vi "HandleScore.vi"(8 "error in (no error)":errorcluster, 11 "Pong in":refnum<class "Pong.lvclass">) -> (0 "error out":errorcluster, 3 "Pong out":refnum<class "Pong.lvclass">)   [LabVIEW 2019, in "RT_Game.lvlib" / "Pong.lvclass"]
uses:
  Pong.lvclass
  C:/Users/FreshBob/Dropbox/VIs/myRIO_GameConsole/RT/RT_Game/Game/Game.lvclass
  Game/Coordinate.ctl
  PongBall/PongBall.lvclass
  C:/Users/FreshBob/Dropbox/VIs/myRIO_GameConsole/RT/RT_Game/GameObject/GameObject.lvclass
  C:/Users/FreshBob/Dropbox/VIs/myRIO_GameConsole/RT/RT_Game/RT_Sprite/RT_Sprite.lvclass
  Game/Game.lvclass/Game.ctl
  GameObject/GameObject.lvclass/GameObject.ctl
  Pong.lvclass/Pong.ctl
  Game/Read Player1Score.vi
  Game/Write Player1Score.vi
  Game/Read Player2Score.vi
  Game/Write Player2Score.vi
  Game/Read Sprite3.vi
  GameObject/Read position.vi
  GameObject/Read size.vi
  Game/Write Sprite3.vi
  RT_Sprite/RT_Sprite.lvclass
  Game/Game.lvclass
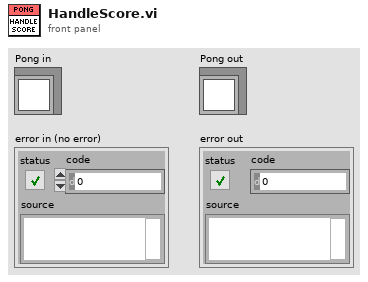
[diagram p1: front panel]
types:
  T1 = typedef "RT_Game.lvlib/Game.lvclass/Coordinate.ctl" = cluster{"x":dbl, "y":dbl}
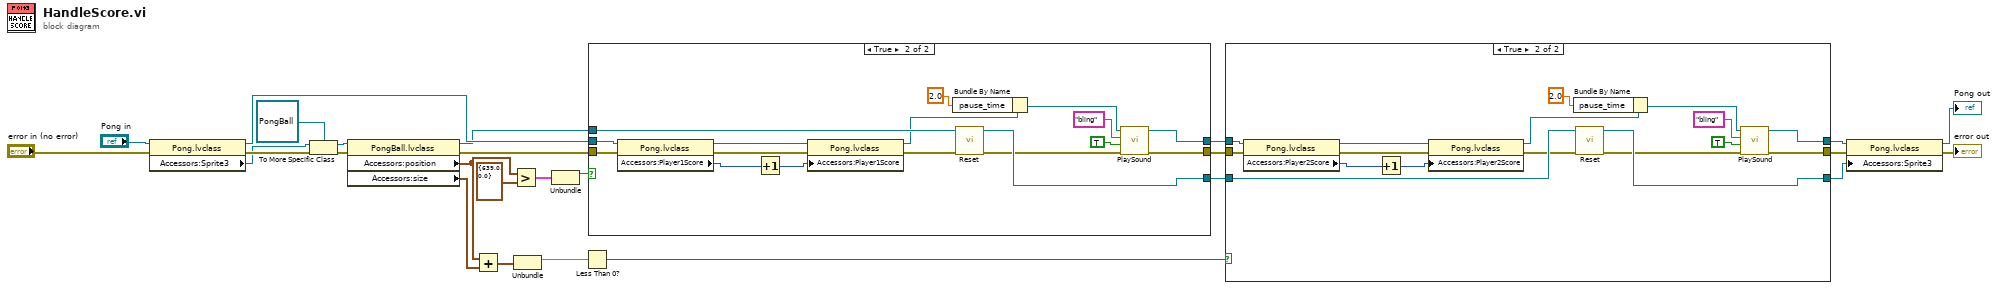
[diagram p0: block diagram]
diagram:
  n1 = property class="Pong.lvclass"(reference="Pong in", error in="error in (no error)") -> (reference out=w11:refnum<class "Pong.lvclass">, error out=w13:errorcluster, "Accessors:Sprite3"=w8:refnum<class "RT_Sprite.lvclass">)
  n2 = To More Specific Class(target class=refnum<class "PongBall.lvclass"> refnum ("RT_Game.lvlib:PongBall.lvclass"), reference=w8, error in=w13) -> (specific class reference=w7:refnum<class "PongBall.lvclass">, error out=w10:errorcluster)
  n3 = property class="PongBall.lvclass"(reference=w7, error in=w10) -> (reference out=w6:refnum<class "PongBall.lvclass">, error out=w22:errorcluster, "Accessors:position"=w17:T1, "Accessors:size"=w21:T1)
  n4 = Add(x=w17, y=w21) -> (x+y=w20:T1)
  n5 = Greater?(x=w17, y=T1 {"x"=639.0, "y"=0.0}) -> (0:w15:cluster{"x":bool, "y":bool})
  n6 = Unbundle(w20) -> ("x"=w19:dbl)  [unwired: 1 out]
  n7 = Unbundle(w15) -> ("x"=w14:bool)  [unwired: 1 out]
  n8 = Less Than 0?(x=w19) -> (x < 0?=w18:bool)
  n9 = case shown="True" w14 {
    tunnel: [w29 w46] -> w26
    tunnel: w11 -> [w29 w40]
    tunnel: w22 -> [w28 w45]
    tunnel: [w28 w44] -> w25
    tunnel: w6 -> [w27 w43]
    tunnel: [w27 w42] -> w2
    frame False {
    }
    frame True {
      n10 = property class="Pong.lvclass"(reference=w40, error in=w45) -> (reference out=w30:refnum<class "Pong.lvclass">, error out=w41:errorcluster, "Accessors:Player1Score"=w39:i32)
      n11 = Increment(x=w39) -> (x+1=w36:i32)
      n12 = property class="Pong.lvclass"(reference=w30, error in=w41, "Accessors:Player1Score"=w36) -> (reference out=w37:refnum<class "Pong.lvclass">, error out=w38:errorcluster)
      n13 = Bundle By Name(cluster=w37, "pause_time"=2.0) -> (w31:refnum<class "Pong.lvclass">)
      n14 = call "Reset.vi"("error in (no error)"=w38, "PongBall in"=w43) -> ("error out"=w34:errorcluster, "PongBall out"=w42:refnum<class "PongBall.lvclass">)  [unwired: 8 in]
      n15 = call "PlaySound.vi"("error in (no error)"=w34, "Overwrite"=TRUE, "Name"="bling", "Game in"=w31) -> ("error out"=w44:errorcluster, "Game out"=w46:refnum<class "Pong.lvclass">)  [unwired: 6 in]
    }
  }
  n16 = case shown="True" w18 {
    tunnel: [w49 w66] -> w4
    tunnel: w26 -> [w49 w61]
    tunnel: w25 -> [w48 w62]
    tunnel: [w48 w65] -> w24
    tunnel: w2 -> [w47 w64]
    tunnel: [w47 w63] -> w1
    frame False {
    }
    frame True {
      n17 = property class="Pong.lvclass"(reference=w61, error in=w62) -> (reference out=w60:refnum<class "Pong.lvclass">, error out=w56:errorcluster, "Accessors:Player2Score"=w59:i32)
      n18 = Increment(x=w59) -> (x+1=w55:i32)
      n19 = property class="Pong.lvclass"(reference=w60, error in=w56, "Accessors:Player2Score"=w55) -> (reference out=w58:refnum<class "Pong.lvclass">, error out=w57:errorcluster)
      n20 = Bundle By Name(cluster=w58, "pause_time"=2.0) -> (w50:refnum<class "Pong.lvclass">)
      n21 = call "Reset.vi"("error in (no error)"=w57, "PongBall in"=w64) -> ("error out"=w51:errorcluster, "PongBall out"=w63:refnum<class "PongBall.lvclass">)  [unwired: 8 in]
      n22 = call "PlaySound.vi"("error in (no error)"=w51, "Overwrite"=TRUE, "Name"="bling", "Game in"=w50) -> ("error out"=w65:errorcluster, "Game out"=w66:refnum<class "Pong.lvclass">)  [unwired: 6 in]
    }
  }
  n23 = property class="Pong.lvclass"(reference=w4, error in=w24, "Accessors:Sprite3"=w1) -> (reference out=→"Pong out":refnum<class "Pong.lvclass">, error out=→"error out":errorcluster)
